vi "登录.vi"() -> ()   [LabVIEW 2018]
uses:
  <vilib>/Utility/config.llb/Write Key (I32).vi
  <vilib>/Utility/config.llb/Read Key (I32).vi
  <vilib>/Utility/config.llb/NI_LVConfig.lvlib
panel:
  out "字符串":string
  in  "复选框":bool
  in  "登录按钮":bool
  in  "密码：":string
  in  "用户名：":string
  # "虚拟数字示波器登录系统"
  # "Virtual Digital Oscilloscope Login System"
  # "用户登录"
  # "登   录"
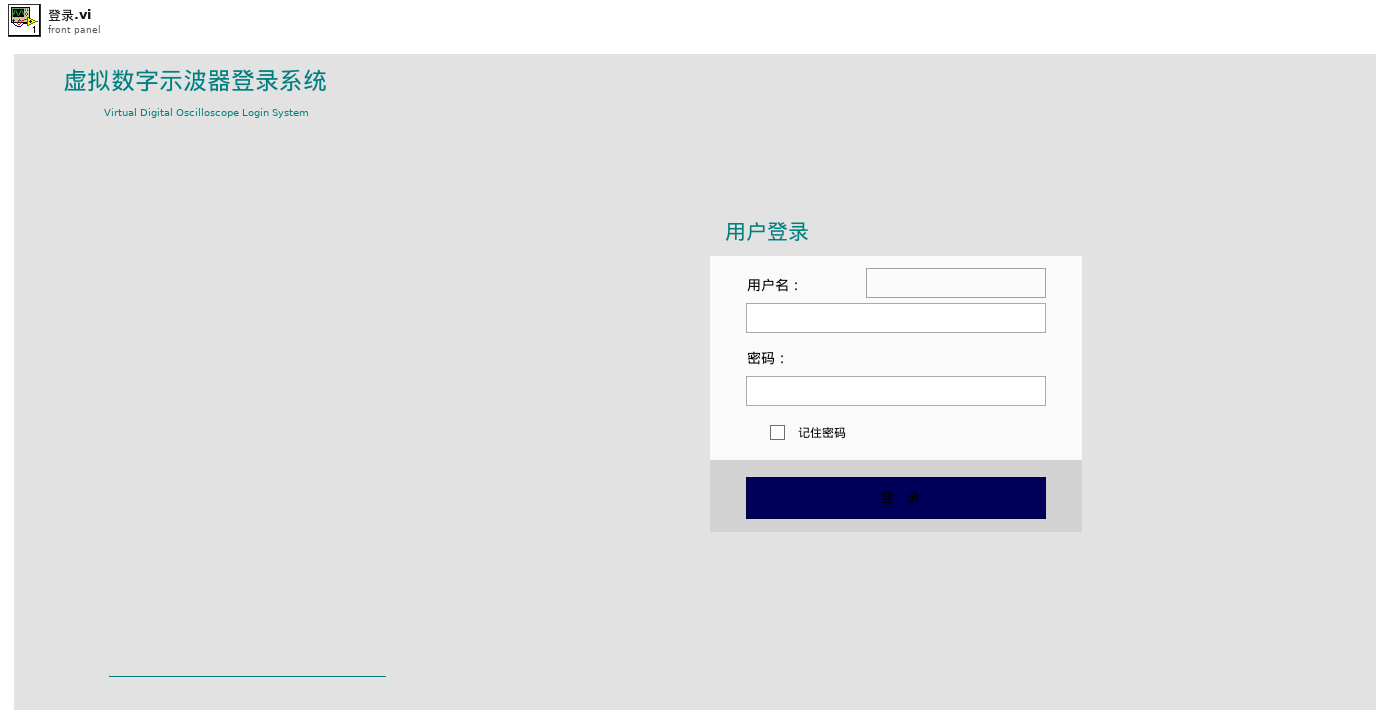
[diagram p1: front panel]
types:
  T1 = typedef "NI_LVConfig.lvlib/Config Data RefNum.ctl" = refnum<k1>
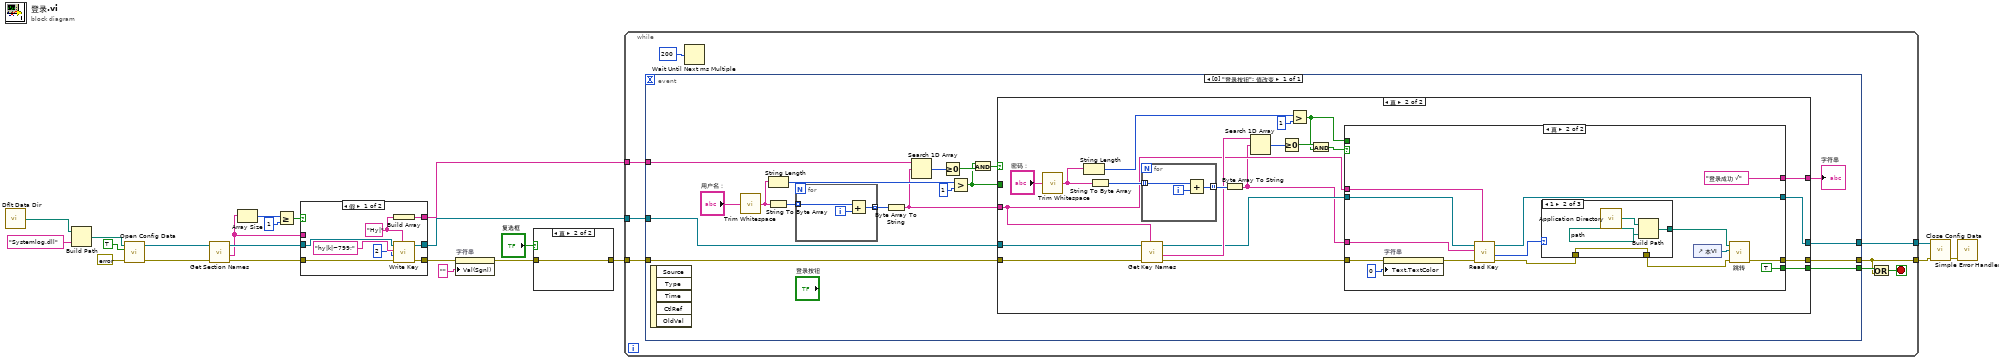
[diagram p0: block diagram]
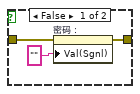
[diagram p3: hidden frame]
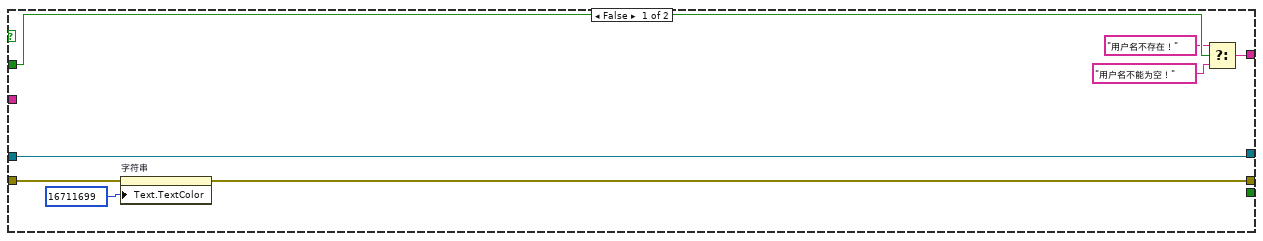
[diagram p4: hidden frame]
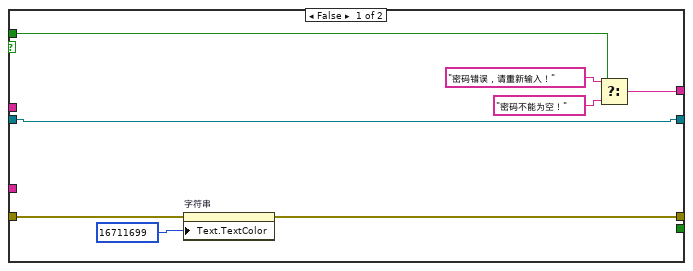
[diagram p5: hidden frame]
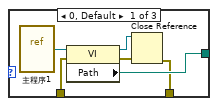
[diagram p6: hidden frame]
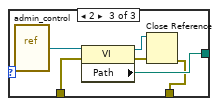
[diagram p7: hidden frame]
diagram:
  n1 = call <vilib>:"Dflt Data Dir.vi"() -> ("App:Default Data Directory"=w16:path)
  n2 = Build Path(base path=w16, name or relative path="Systemlog.dll" ("pattern (all files)")) -> (appended path=w17:path)
  n3 = call <vilib>:"Open Config Data.vi"("error in (no error)"=errorcluster {"status"=FALSE, "code"=0, "source"=""} ("错误输入（无错误）"), "create file if necessary (T)"=TRUE, "configuration file path"=w17) -> ("error out"=w19:errorcluster, "refnum"=w18:T1)  [unwired: 6 in, 1 out]
  n4 = call <vilib>:"Get Section Names.vi"("error in (no error)"=w19, "refnum"=w18) -> ("error out"=w5:errorcluster, "section names"=w2:string[], "refnum out"=w6:T1)  [unwired: 7 in]
  n5 = Array Size(array=w2) -> (size(s)=w9:i32)
  n6 = Greater Or Equal?(x=w9, y=1) -> (x >= y?=w7:bool)
  n7 = case shown="假" w7 {
    tunnel: w6 -> [w31 w34]
    tunnel: w5 -> [w30 w33]
    tunnel: [w29 w34] -> w4
    tunnel: [w28 w33] -> w3
    tunnel: w2 -> [_ w32]
    tunnel: [w24 w32] -> w1
    frame False {
      w25 = "Hy|" ("section")
      n8 = Build Array(w25) -> (w24:string[])
      n9 = call-poly <vilib>:"Write Key.vi"("section"=w25, "error in (no error)"=w30, "value"=2, "key"="hy|k|~799;", "refnum"=w31) -> ("error out"=w28:errorcluster, "refnum out"=w29:T1)  [unwired: 4 in, 1 out]
    }
    frame True {
    }
  }
  n10 = property on="字符串" class="Str"(error in=w3, "Val(Sgnl)"="" ("值(信号)")) -> (error out=w21:errorcluster)  [unwired: 1 in, 1 out]
  n11 = case shown="真" "复选框" {
    tunnel: w21 -> [w37 w38]
    tunnel: [w36 w38] -> w20
    frame False {
      n12 = property on="密码：" class="Str"(error in=w37, "Val(Sgnl)"="" ("值(信号)")) -> (error out=w36:errorcluster)  [unwired: 1 in, 1 out]
    }
    frame True {
    }
  }
  n13 = while {
    tunnel: w20 -> [w43]
    tunnel: w4 -> [w41]
    tunnel: w1 -> [w42]
    tunnel: [w40] -> w12
    tunnel: [w39] -> w11
    stop <- w44 stop-if-true
    n14 = event shown="[0] \"登录按钮\": 值改变" {
      selector: _ -> [_]
      dyn-events: _ -> [_]
      timeout: _ -> [_]
      tunnel: [w64] -> w45
      tunnel: w43 -> [w63]
      tunnel: [w62] -> w39
      tunnel: w42 -> [w57]
      tunnel: w41 -> [w48]
      tunnel: [w47] -> w40
      event "登录按钮": Value Change {
        n15 = event-data() -> ()  [unwired: 1 in, 5 out]
        n16 = call <vilib>:"Trim Whitespace.vi"("string"="用户名：") -> ("trimmed string"=w56:string)  [unwired: 1 in]
        n17 = String Length(string=w56) -> (length=w55:i32)
        n18 = String To Byte Array(string=w56) -> (unsigned byte array=w59:u8[])
        n19 = for {
          tunnel: w59 -> [w66] mode=indexing
          tunnel: [w65] -> w58 mode=indexing
          i -> [w67]
          n20 = Add(x=w66, y=w67) -> (x+y=w65:i32)
        }
        n21 = Byte Array To String(unsigned byte array=w58) -> (string=w50:string)
        n22 = Search 1D Array(1D array=w57, element=w50) -> (index of element=w53:i32)  [unwired: 1 in]
        n23 = Greater Or Equal To 0?(x=w53) -> (x >= 0?=w52:bool)
        n24 = Greater?(x=w55, y=1) -> (0:w49:bool)
        n25 = And(x=w49, y=w52) -> (x .and. y?=w51:bool)
        n26 = case shown="真" w51 {
          tunnel: [w75 w96] -> w61
          tunnel: [_ w95] -> w64
          tunnel: w63 -> [w74 w92]
          tunnel: [w73 w94] -> w62
          tunnel: w50 -> [_ w77]
          tunnel: w49 -> [w71 _]
          tunnel: w48 -> [w68 w93]
          tunnel: [w68 w79] -> w47
          frame False {
            n27 = property on="字符串" class="Str"(error in=w74, "Text.TextColor"=u32 16711699 ("文本.文本颜色:文本颜色")) -> (error out=w73:errorcluster)  [unwired: 1 in, 1 out]
            n28 = Select(t="用户名不存在！", s=w71, f="用户名不能为空！") -> (s? t:f=w75:string)
          }
          frame True {
            n29 = call <vilib>:"Trim Whitespace.vi"("string"="密码：") -> ("trimmed string"=w88:string)  [unwired: 1 in]
            n30 = String Length(string=w88) -> (length=w89:i32)
            n31 = String To Byte Array(string=w88) -> (unsigned byte array=w87:u8[])
            n32 = for {
              tunnel: w87 -> [w98] mode=indexing
              tunnel: [w97] -> w86 mode=indexing
              i -> [w99]
              n33 = Add(x=w98, y=w99) -> (x+y=w97:i32)
            }
            n34 = call <vilib>:"Get Key Names.vi"("section"=w77, "error in (no error)"=w92, "refnum"=w93) -> ("error out"=w82:errorcluster, "key names"=w85:string[], "refnum out"=w80:T1)  [unwired: 5 in, 1 out]
            n35 = Byte Array To String(unsigned byte array=w86) -> (string=w76:string)
            n36 = Search 1D Array(1D array=w85, element=w76) -> (index of element=w84:i32)  [unwired: 1 in]
            n37 = Greater Or Equal To 0?(x=w84) -> (x >= 0?=w81:bool)
            n38 = Greater?(x=w89, y=1) -> (0:w78:bool)
            n39 = And(x=w81, y=w78) -> (x .and. y?=w83:bool)
            n40 = case shown="真" w83 {
              tunnel: [w107 "登录成功 √"] -> w96
              tunnel: [_ TRUE] -> w95
              tunnel: w82 -> [w105 w115]
              tunnel: [w104 w119] -> w94
              tunnel: w78 -> [w103 _]
              tunnel: w80 -> [w100 w116]
              tunnel: [w100 w111] -> w79
              tunnel: w77 -> [_ w113]
              tunnel: w76 -> [_ w112]
              frame False {
                n41 = property on="字符串" class="Str"(error in=w105, "Text.TextColor"=u32 16711699 ("文本.文本颜色:文本颜色")) -> (error out=w104:errorcluster)  [unwired: 1 in, 1 out]
                n42 = Select(t="密码错误，请重新输入！", s=w103, f="密码不能为空！") -> (s? t:f=w107:string)
              }
              frame True {
                n43 = property on="字符串" class="Str"(error in=w115, "Text.TextColor"=u32 0 ("文本.文本颜色:文本颜色")) -> (error out=w114:errorcluster)  [unwired: 1 in, 1 out]
                n44 = call-poly <vilib>:"Read Key.vi"("section"=w113, "error in (no error)"=w114, "key"=w112, "refnum"=w116) -> ("error out"=w109:errorcluster, "value"=w110:i32, "refnum out"=w111:T1)  [unwired: 4 in, 1 out]
                n45 = case shown="1" w110 {
                  tunnel: [w127 w131 w135] -> w117
                  tunnel: w109 -> [w124 w130 w136]
                  tunnel: [w123 w130 w133] -> w108
                  frame 0, Default {
                    n46 = vi-ref "主程序1.vi"() -> (w128:refnum<vi>)
                    n47 = property class="VI"(reference=w128, error in=w124) -> (reference out=w125:refnum<vi>, error out=w126:errorcluster, "Path"=w127:path)
                    n48 = Close Reference(reference=w125, error in (no error)=w126) -> (error out=w123:errorcluster)
                  }
                  frame 1 {
                    n49 = call <vilib>:"Application Directory.vi"() -> ("Application Directory"=w132:path)
                    n50 = Build Path(base path=w132, name or relative path=path "登录/主程序1.vi") -> (appended path=w131:path)
                  }
                  frame 2 {
                    n51 = vi-ref "admin_control.vi"() -> (w134:refnum<vi>)
                    n52 = property class="VI"(reference=w134, error in=w136) -> (reference out=w137:refnum<vi>, error out=w138:errorcluster, "Path"=w135:path)
                    n53 = Close Reference(reference=w137, error in (no error)=w138) -> (error out=w133:errorcluster)
                  }
                }
                n54 = control-ref of="本VI"() -> (w120:refnum<vi>)
                n55 = call "跳转.vi"("错误输入（无错误）"=w108, "引用"=w120, "路径"=w117) -> ("错误输出"=w119:errorcluster)  [unwired: 8 in]
              }
            }
          }
        }
        "字符串" <- w61
      }
    }
    n56 = Wait Until Next ms Multiple(millisecond multiple=u32 200 ("毫秒倍数")) -> ()  [unwired: 1 out]
    n57 = Or(x=w45, y=w39) -> (x .or. y?=w44:bool)
  }
  n58 = call <vilib>:"Close Config Data.vi"("error in (no error)"=w11, "refnum"=w12) -> ("error out"=w10:errorcluster)  [unwired: 8 in, 1 out]
  n59 = call <vilib>:"Simple Error Handler.vi"("error in (no error)"=w10) -> ()  [unwired: 4 in, 5 out]
